vi "calculate score.vi"(9 "note count":i32, 10 "max combo":i32, 11 "note acc":i32[](array[numeric])) -> (1 "accuracy":dbl, 3 "score":i32)   [LabVIEW 2023]
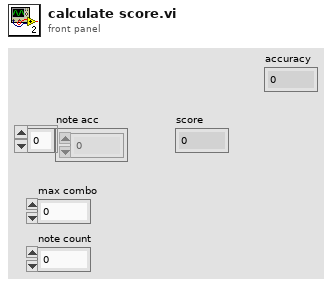
[diagram p1: front panel]
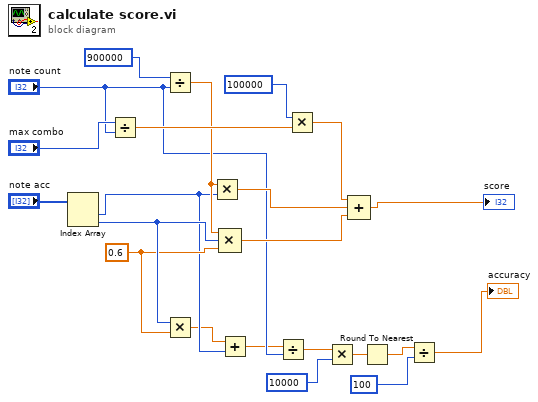
[diagram p0: block diagram]
diagram:
  w11 = 0.6
  n1 = Index Array(array="note acc") -> (element #1=w10:i32, element #2=w12:i32)  [unwired: 2 in]
  n2 = Divide(x="max combo", y="note count") -> (x/y=w19:dbl)
  n3 = Divide(x=900000, y="note count") -> (x/y=w16:dbl)
  n4 = Multiply(x=w12, y=w11) -> (x*y=w9:dbl)
  n5 = Multiply(x=w16, y=w10) -> (x*y=w20:dbl)
  n6 = Compound Arithmetic op=MULTIPLY(w16, w12, w11) -> (w15:dbl)
  n7 = Add(x=w9, y=w10) -> (x+y=w7:dbl)
  n8 = Divide(x=w7, y="note count") -> (x/y=w5:dbl)
  n9 = Multiply(x=100000, y=w19) -> (x*y=w17:dbl)
  n10 = Multiply(x=w5, y=10000) -> (x*y=w4:dbl)
  n11 = Compound Arithmetic op=ADD(w17, w20, w15) -> (→"score":dbl)
  n12 = Round To Nearest(number=w4) -> (nearest integer value=w3:dbl)
  n13 = Divide(x=w3, y=100) -> (x/y=→"accuracy":dbl)
